vi "CLD 11Unbundle data SubVI.vi"(8 "Fehler (Eingang, kein Fehler)":errorcluster, 10 "Nr. des aktuellen Zustands":i32, 11 "[Daten, Eingang]":T1[](array[typedef])) -> (0 "Fehler (Ausgang)":errorcluster, 1 "Zustand 3":bool, 2 "Zustand 2":bool, 3 "[Daten, Ausgang]":T1[](array[typedef]), 4 "Nächste Verweildauer":dbl, 5 "Zustand 1":bool, 6 "Verweildauer":dbl)   [LabVIEW 2009]
doc: "CLD 11 - Utility zum Aufschlüsseln von Daten. Kopiert von CLD-Lösung 10."
uses:
  CLD 11 CSV file data structure.ctl
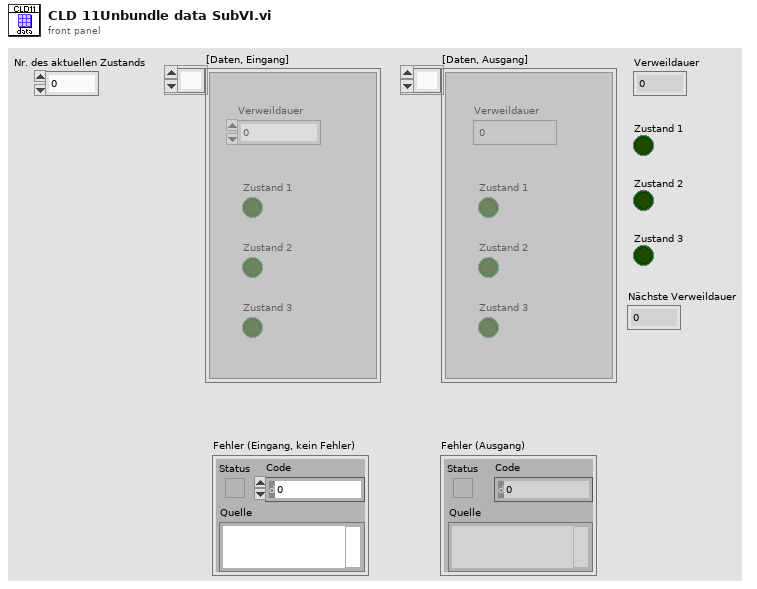
[diagram p1: front panel]
types:
  T1 = typedef "CLD 11 CSV file data structure.ctl" = cluster{"Verweildauer":i32, "Zustand 1":bool, "Zustand 2":bool, "Zustand 3":bool}
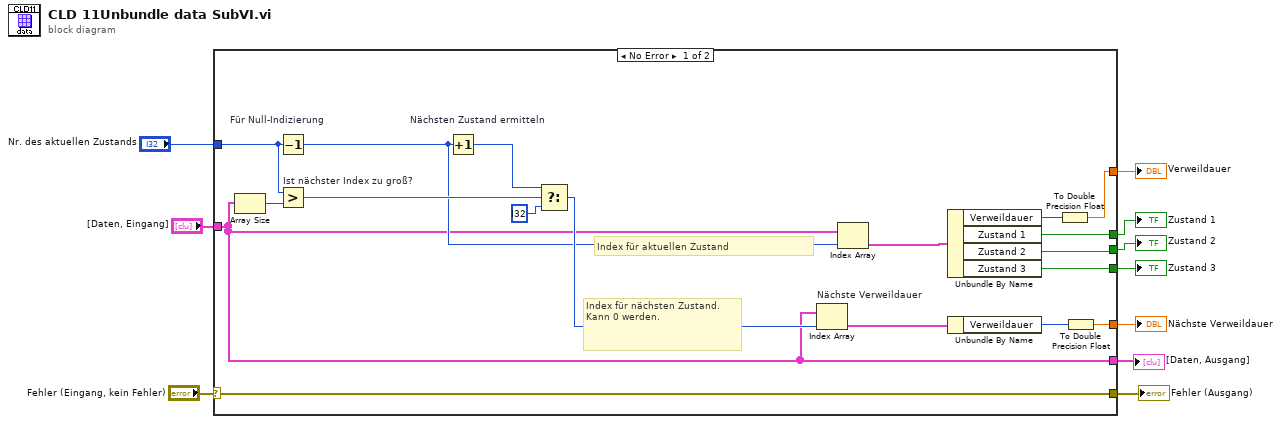
[diagram p0: block diagram]
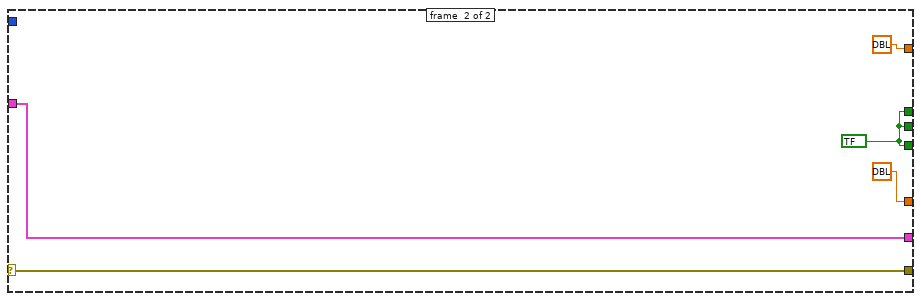
[diagram p2: hidden frame]
diagram:
  n1 = case shown="No Error" "Fehler (Eingang, kein Fehler)" {
    selector: "Fehler (Eingang, kein Fehler)" -> [w16 w31]
    tunnel: [w26 dbl ?] -> w10
    tunnel: "[Daten, Eingang]" -> [w12 w29]
    tunnel: [w18 dbl ?] -> w8
    tunnel: [w16 w31] -> w6
    tunnel: [w15 w30] -> w5
    tunnel: [w14 w30] -> w4
    tunnel: [w13 w30] -> w3
    tunnel: [w12 w29] -> w2
    tunnel: "Nr. des aktuellen Zustands" -> [w11 _]
    frame #0 {
      # "Index für nächsten Zustand. Kann 0 werden."
      # "Index für aktuellen Zustand"
      n2 = Array Size(array=w12) -> (size(s)=w22:i32)
      n3 = Decrement "Für Null-Indizierung"(x=w11) -> (x-1=w17:i32)
      n4 = Greater? "Ist nächster Index zu groß?"(x=w11, y=w22) -> (0:w25:bool)
      n5 = Increment "Nächsten Zustand ermitteln"(x=w17) -> (x+1=w21:i32)
      n6 = Select(t=w21, s=w25, f=i32 ?) -> (s? t:f=w23:i32)
      n7 = Index Array "Nächste Verweildauer"(array=w12, index=w23) -> (element=w20:T1)
      n8 = Index Array(array=w12, index=w17) -> (element=w28:T1)
      n9 = Unbundle By Name(w28) -> ("Verweildauer"=w27:i32, "Zustand 1"=w15:bool, "Zustand 2"=w14:bool, "Zustand 3"=w13:bool)
      n10 = Unbundle By Name(w20) -> ("Verweildauer"=w19:i32)
      n11 = To Double Precision Float(number=w27) -> (double precision float=w26:dbl)
      n12 = To Double Precision Float(number=w19) -> (double precision float=w18:dbl)
    }
    frame #1 {
      w30 = bool ? ("Zustand 1")
    }
  }
  "Verweildauer" <- w10
  "Nächste Verweildauer" <- w8
  "Fehler (Ausgang)" <- w6
  "Zustand 1" <- w5
  "Zustand 2" <- w4
  "Zustand 3" <- w3
  "[Daten, Ausgang]" <- w2
